vi "Get Coverage for All Executed VIs.vi"(8 "error in (no error)":errorcluster, 11 "Coverage Analyzer in":refnum<class "Coverage Analyzer.lvclass">) -> (0 "error out":errorcluster, 2 "Code Coverage":map{path, dbl}(c390), 3 "Coverage Analyzer out":refnum<class "Coverage Analyzer.lvclass">)   [LabVIEW 2020, in "Coverage Analyzer.lvclass"]
uses:
  Coverage Analyzer.lvclass
  Coverage Analyzer.lvclass/Coverage Analyzer.ctl
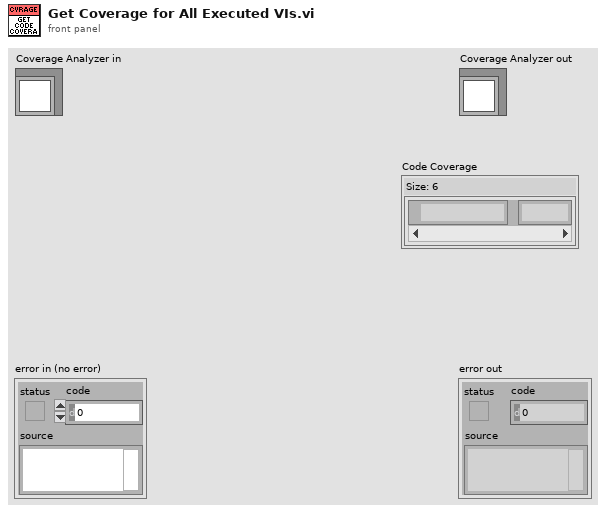
[diagram p1: front panel]
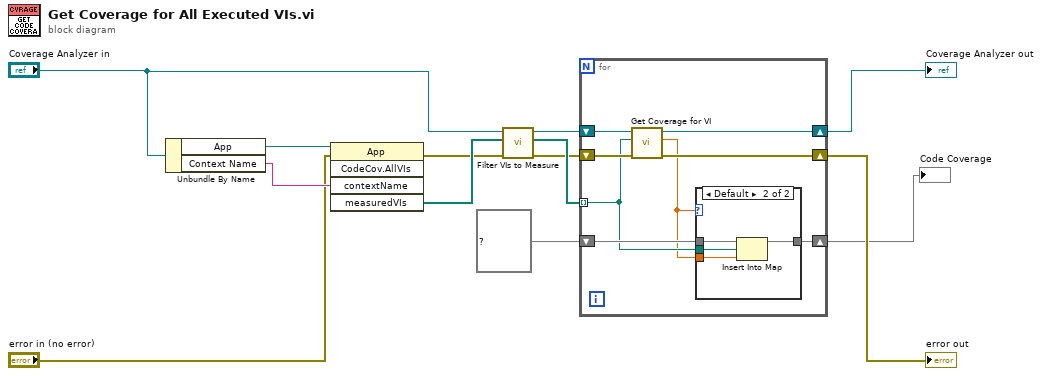
[diagram p0: block diagram]
diagram:
  n1 = Unbundle By Name("Coverage Analyzer in") -> ("App"=w12:refnum<vi>, "Context Name"=w13:string)
  n2 = invoke class="App" method="CodeCov.AllVIs"(reference=w12, error in="error in (no error)", "contextName"=w13) -> (error out=w2:errorcluster, "measuredVIs"=w4:path[])  [unwired: 2 in, 3 out]
  n3 = call "Filter VIs to Measure.vi"("error in (no error)"=w2, "VI Paths"=w4, "Coverage Analyzer in"="Coverage Analyzer in") -> ("error out"=w1:errorcluster, "Filtered VI Paths"=w3:path[], "Coverage Analyzer out"=w5:refnum<class "Coverage Analyzer.lvclass">)  [unwired: 6 in]
  n4 = for {
    shift-right: [w20] -> w11
    shift-left: w5 -> [w21]
    shift-right: [w18] -> w9
    shift-left: w1 -> [w19]
    tunnel: w3 -> [w15] mode=indexing
    shift-right: [w16] -> w7
    shift-left: map{path, dbl} {} ("Code Coverage") -> [w17]
    n5 = call "Get Coverage for VI.vi"("error in (no error)"=w19, "VI Path"=w15, "Coverage Analyzer in"=w21) -> ("error out"=w18:errorcluster, "Percentage"=w14:dbl, "Coverage Analyzer out"=w20:refnum<class "Coverage Analyzer.lvclass">)  [unwired: 5 in, 1 out]
    n6 = case shown="Default" w14 {
      tunnel: w17 -> [w22 w26]
      tunnel: [w22 w25] -> w16
      tunnel: w14 -> [_ w24]
      tunnel: w15 -> [_ w23]
      frame 0 {
      }
      frame Default {
        n7 = Insert Into Map(map in=w26, key=w23, value=w24) -> (map out=w25:map{path, dbl})  [unwired: 2 out]
      }
    }
  }
  "error out" <- w9
  "Coverage Analyzer out" <- w11
  "Code Coverage" <- w7
